vi "Update Offgrid VF Device.vi"(6 "Reset Swap Delay":bool, 7 "Global Configuration":T1={"Microgrid ID"=1, "VF Device ID"="", "Ongrid VF Priority"=[], "Offgrid VF Priority"=[], "AutoSwap Offgrid VF"=0, "AutoSwap Offgrid VF Delay (sec)"=0.0, "AutoSwap Resynch VF"=0, "PCC Device ID"="", "Device ID Array"=[], "Nominal Voltage"=0.0, "Nominal Frequency"=0.0, "Resynch Timeout (sec)"=0.0, "Island VF Activate Timeout (sec)"=90.0, "Island PCC Target Power (kW)"=0.0, "Island PCC Target Power Timeout (sec)"=0.0, "Island Grid Settle Time (sec)"=0.0, "Island PCC Failure Timeout (sec)"=0.0, "Activation Devices Present Timeout (sec)"=0.0, "Activation Devices Activated Timeout (sec)"=0.0, "Blackstart VF GenMode Wait (sec)"=0.0, "Blackstart VF DERCtrl Wait (sec)"=0.0, "Blackstart Success Wait (sec)"=0.0, "OnGrid Optimization Delay (sec)"=0.0, "OffGrid Optimization Delay (sec)"=0.0, "Resynch Frequency (Hz)"=0.0, "Optimization Path"=""}, 8 "error in":errorcluster, 11 "Off-Grid in":refnum<class "Off-Grid.lvclass">) -> (0 "error out":errorcluster, 3 "Off-Grid out":refnum<class "Off-Grid.lvclass">)   [LabVIEW 2018, in "Off-Grid Actor.lvlib" / "Off-Grid.lvclass"]
uses:
  Off-Grid.lvclass
  C:/Users/Administrator/Desktop/LabVIEW EMS/EMS Generic Actor/EMS Generic/EMS Generic.lvclass
  C:/Users/Administrator/Desktop/LabVIEW EMS/Device Communication and Control Abstract Actor/Device Communication and Control Abstract/Device Communication and Control Abstract.lvclass
  EMS Generic Actor/EMS Generic/Controls/Global Configuration.ctl
  <vilib>/ORNL/CSEISMIC DDS/CSEISMIC DDS Base/Data Types/Controls/DeviceID.ctl
  EMS Generic Actor/EMS Generic/EMS Generic.lvclass/EMS Generic.ctl
  <vilib>/ORNL/CSEISMIC DDS/CSEISMIC DDS Base/Data Types/DER_VF.ctl
  <vilib>/ActorFramework/Actor/Actor.lvclass/Actor.ctl
  Device Communication and Control Abstract Actor/Device Communication and Control Abstract/Device Communication and Control Abstract.lvclass/Device Communication and Control Abstract.ctl
  Device Communication and Control Abstract Actor/Device Communication and Control Abstract Messages/Set DER VF Msg/Set DER VF Msg.lvclass/Set DER VF Msg.ctl
  <vilib>/ActorFramework/Message Enqueuer/Message Enqueuer.lvclass/Message Enqueuer.ctl
  EMS Generic Actor/EMS Generic/Accessors - Global Configuration/Read Global Configuration.vi
  Device Communication and Control Abstract Actor/Device Communication and Control Abstract Messages/Set DER VF Msg/Send Set DER VF.vi
  <vilib>/ActorFramework/Actor/Read Caller Enqueuer.vi
  <vilib>/ActorFramework/Message Enqueuer/Enqueue.vi
  Device Communication and Control Abstract Actor/Device Communication and Control Abstract/Device Communication and Control Abstract.lvclass
  C:/Program Files (x86)/National Instruments/LabVIEW 2018/vi.lib/ActorFramework/Actor/Actor.lvclass
  Device Communication and Control Abstract Actor/Device Communication and Control Abstract Messages/Set DER VF Msg/Set DER VF Msg.lvclass
  C:/Program Files (x86)/National Instruments/LabVIEW 2018/vi.lib/ActorFramework/Message/Message.lvclass
  EMS Generic Actor/EMS Generic/Accessors - Global Configuration/Update Global Configuration.vi
  <vilib>/ActorFramework/Message Priority Queue/Priority Enqueue.vi
  EMS Generic Actor/EMS Generic/EMS Generic.lvclass
  <vilib>/ORNL/CSEISMIC DDS/CSEISMIC DDS Base/CSEISMIC DDS.lvclass
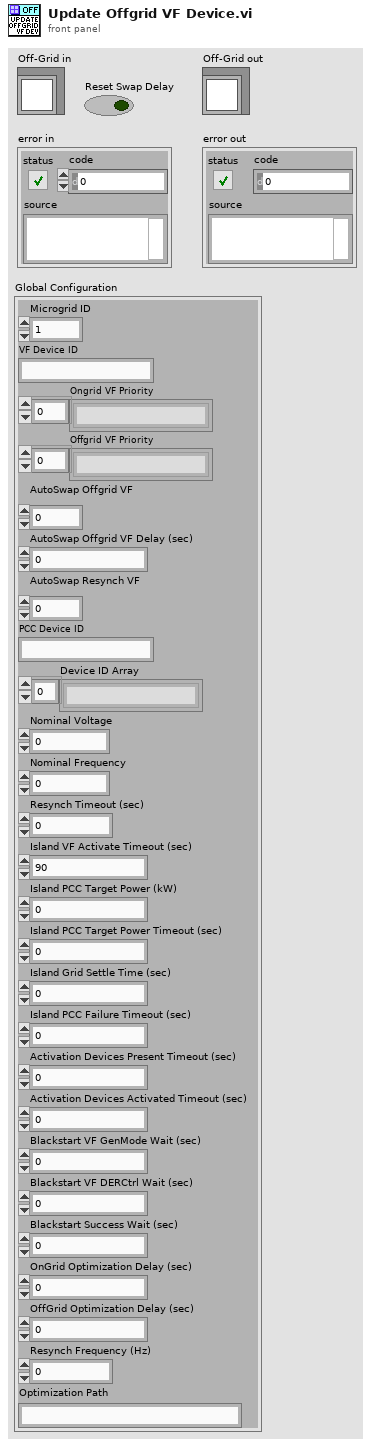
[diagram p1: front panel]
types:
  T1 = typedef "EMS Generic Actor.lvlib/EMS Generic.lvclass/Global Configuration.ctl" = cluster{"Microgrid ID":u8, "VF Device ID":T2, "Ongrid VF Priority":T2[], "Offgrid VF Priority":T2[], "AutoSwap Offgrid VF":u32, "AutoSwap Offgrid VF Delay (sec)":dbl, "AutoSwap Resynch VF":u32, "PCC Device ID":T2, "Device ID Array":T2[], "Nominal Voltage":dbl, "Nominal Frequency":dbl, "Resynch Timeout (sec)":dbl, "Island VF Activate Timeout (sec)":dbl, "Island PCC Target Power (kW)":dbl, "Island PCC Target Power Timeout (sec)":dbl, "Island Grid Settle Time (sec)":dbl, "Island PCC Failure Timeout (sec)":dbl, "Activation Devices Present Timeout (sec)":dbl, "Activation Devices Activated Timeout (sec)":dbl, "Blackstart VF GenMode Wait (sec)":dbl, "Blackstart VF DERCtrl Wait (sec)":dbl, "Blackstart Success Wait (sec)":dbl, "OnGrid Optimization Delay (sec)":dbl, "OffGrid Optimization Delay (sec)":dbl, "Resynch Frequency (Hz)":dbl, "Optimization Path":string}
  T2 = typedef "CSEISMIC DDS.lvlib/CSEISMIC DDS.lvclass/DeviceID.ctl" = string
  T3 = typedef "CSEISMIC DDS.lvlib/CSEISMIC DDS.lvclass/DER_VF.ctl" = cluster{"DeviceID":T2}
  T4 = typedef "EMS Generic Actor.lvlib/EMS Generic.lvclass/Data Type DVRs.ctl" = cluster{"IED_Status":refnum<data-value>, "IED_Status_0":refnum<data-value>, "DER_Measurement":refnum<data-value>, "DER_Info":refnum<data-value>, "DER_Status":refnum<data-value>, "ES_Measurement":refnum<data-value>, "ES_Info":refnum<data-value>, "PV_Info":refnum<data-value>, "SmartRelay_Info":refnum<data-value>, "SmartRelay_Measurement":refnum<data-value>, "Meter_Info":refnum<data-value>, "Meter_Measurement":refnum<data-value>, "HVAC_Status":refnum<data-value>, "HVAC_Measurement":refnum<data-value>, "PriceData_RealTime":refnum<data-value>, "PriceData_Demand":refnum<data-value>, "PriceData_Energy":refnum<data-value>, "ForecastData_Long":refnum<data-value>, "ForecastData_Short":refnum<data-value>, "DER_Control":refnum<data-value>, "DER_SetPointF":refnum<data-value>, "DER_SetPointP":refnum<data-value>, "DER_SetPointQ":refnum<data-value>, "DER_SetPointPF":refnum<data-value>, "DER_SetPointV":refnum<data-value>, "PV_setCurtailment":refnum<data-value>, "PV_setRampRate":refnum<data-value>, "Relay_Control":refnum<data-value>, "Load_Control":refnum<data-value>, "HVAC_Control":refnum<data-value>, "Generator_Info":refnum<data-value>, "ForecastData_Long_Backup":refnum<data-value>, "PriceData_RealTime_Backup":refnum<data-value>}
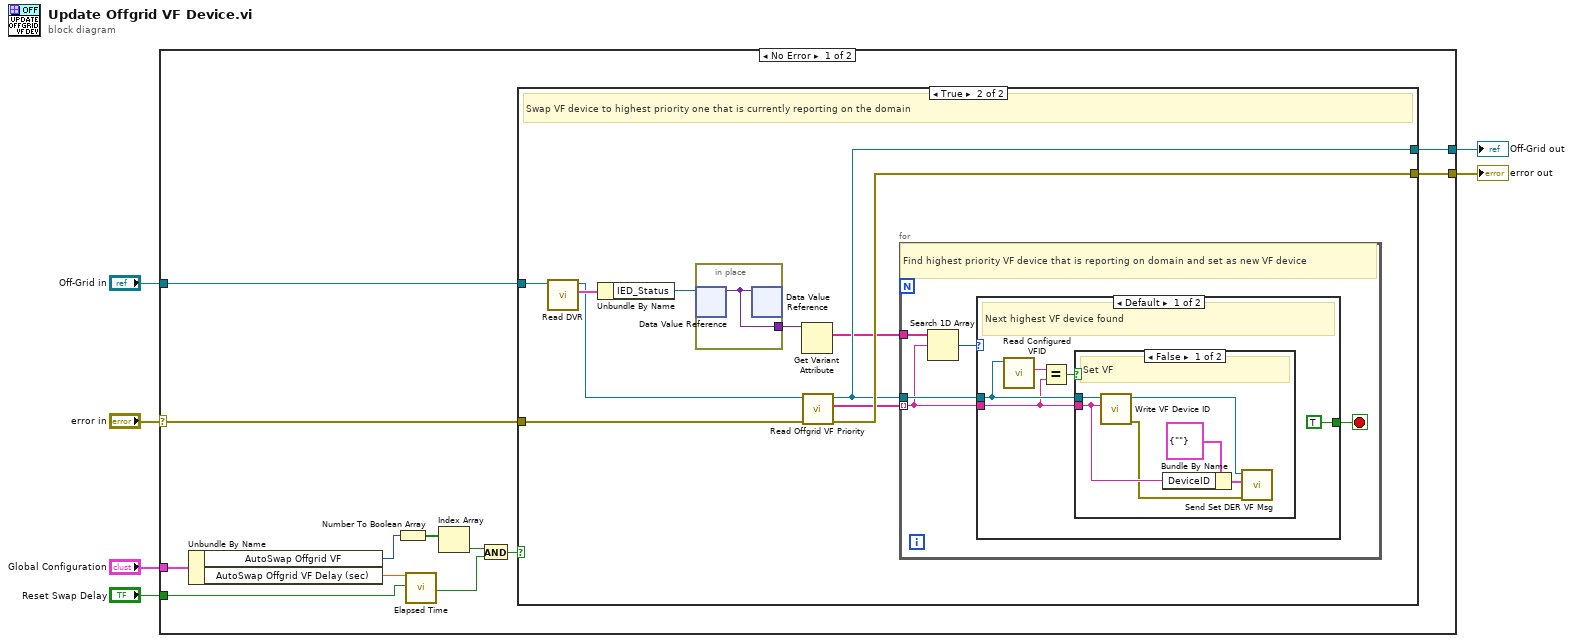
[diagram p0: block diagram]
diagram:
  n1 = case shown="No Error" "error in" {
    selector: "error in" -> [w15 w48]
    tunnel: [w18 w49] -> w6
    tunnel: "Off-Grid in" -> [w17 w49]
    tunnel: [w16 w48] -> w4
    tunnel: "Global Configuration" -> [w14 _]
    tunnel: "Reset Swap Delay" -> [w12 _]
    frame No Error {
      n2 = Unbundle By Name(w14) -> ("AutoSwap Offgrid VF"=w9:u32, "AutoSwap Offgrid VF Delay (sec)"=w13:dbl)
      n3 = Number To Boolean Array(number=w9) -> (Boolean array=w8:bool[])
      n4 = call "Elapsed Time"("Time Target (s)"=w13, "Reset"=w12) -> ("Time has Elapsed"=w11:bool)  [unwired: 10 in, 7 out]
      n5 = Index Array(array=w8) -> (element=w7:bool)  [unwired: 1 in]
      n6 = And(x=w7, y=w11) -> (x .and. y?=w10:bool)
      n7 = case shown="True" w10 {
        tunnel: [w20 w26] -> w18
        tunnel: w17 -> [w20 w22]
        tunnel: [w19 w30] -> w16
        tunnel: w15 -> [w19 w29]
        frame False {
          # "Either we're not auto swapping or it's not yet time to swap.  Do nothing."
        }
        frame True {
          # "Swap VF device to highest priority one that is currently reporting on the domain"
          n8 = call "Read DVR.vi"("EMS Generic in"=w22) -> ("DVR"=w28:T4, "EMS Generic out"=w21:refnum<class "Off-Grid.lvclass">)  [unwired: 9 in]
          n9 = Unbundle By Name(w28) -> ("IED_Status"=w25:refnum<data-value>)
          n10 = in-place {
            in-place-border: [w31] -> w24
            n11 = in-place-dvr #1(w25) -> (w31:variant)  [unwired: 1 out]
            n12 = in-place-dvr #1(w31) -> ()  [unwired: 2 out]
          }
          n13 = Get Variant Attribute(Variant=w24) -> (names=w23:string[])  [unwired: 3 in, 3 out]
          n14 = call "Read Offgrid VF Priority.vi"("error in"=w29, "EMS Generic in"=w21) -> ("error out"=w30:errorcluster, "Offgrid VF Priority"=w27:T2[], "EMS Generic out"=w26:refnum<class "Off-Grid.lvclass">)  [unwired: 7 in]
          n15 = for {
            tunnel: w27 -> [w33] mode=indexing
            tunnel: w23 -> [w36]
            tunnel: w26 -> [w34]
            stop <- w32 stop-if-true
            # "Find highest priority VF device that is reporting on domain and set as new VF device"
            n16 = Search 1D Array(1D array=w36, element=w33) -> (index of element=w35:i32)  [unwired: 1 in]
            n17 = case shown="Default" w35 {
              tunnel: w34 -> [w40 _]
              tunnel: w33 -> [w38 _]
              tunnel: [TRUE _] -> w32
              frame Default {
                # "Next highest VF device found"
                n18 = call "Read Configured VFID.vi"("EMS Generic in"=w40) -> ("VFID"=w39:T2)  [unwired: 8 in, 2 out]
                n19 = Equal?(x=w39, y=w38) -> (x = y?=w37:bool)
                n20 = case shown="False" w37 {
                  tunnel: w38 -> [w44 _]
                  tunnel: w40 -> [w47 _]
                  frame False {
                    # "Set VF"
                    n21 = call "Write VF Device ID.vi"("VF Device"=w44, "EMS Generic in"=w47) -> ("error out"=w43:errorcluster, "EMS Generic out"=w42:refnum<class "Off-Grid.lvclass">)  [unwired: 8 in]
                    n22 = Bundle By Name(cluster=T3 {"DeviceID"=""} ("DER_VF"), "DeviceID"=w44) -> (w45:T3)
                    n23 = call "Send Set DER VF Msg.vi"("error in"=w43, "DER_VF"=w45, "SCADA Sub Abstract in"=w42) -> ()  [unwired: 7 in, 2 out]
                  }
                  frame True {
                    # "Already VF"
                  }
                }
              }
              frame -1 {
                # "Backup VF device not reporting on domain"
              }
            }
          }
        }
      }
    }
    frame Error {
    }
  }
  "Off-Grid out" <- w6
  "error out" <- w4
